vi "Update Position.vi"(6 "Upper Boundary":i16, 7 "Lower Boundary":dbl, 8 "Hit Lower Boundary?":bool, 9 "Hit Upper Boundary?":bool, 10 "Velocity":dbl, 11 "Position":dbl) -> (3 "Updated Position":dbl)   [LabVIEW 2015]
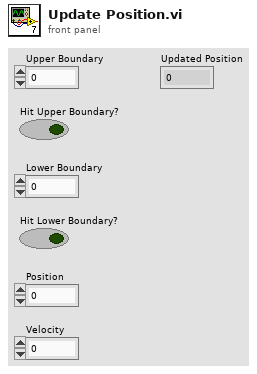
[diagram p1: front panel]
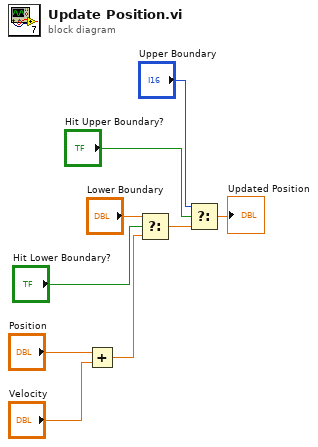
[diagram p0: block diagram]
diagram:
  n1 = Add(x="Position", y="Velocity") -> (x+y=w5:dbl)
  n2 = Select(t="Lower Boundary", s="Hit Lower Boundary?", f=w5) -> (s? t:f=w8:dbl)
  n3 = Select(t="Upper Boundary", s="Hit Upper Boundary?", f=w8) -> (s? t:f=→"Updated Position":dbl)
